vi "LabviewChat.vi"() -> ()   [LabVIEW 2015]
panel:
  out "error 2":errorcluster
  in  "Their IP Address":string
  in  "Receive Port":u16=20090
  in  "Send Port":u16=20090
  in  "Send":bool
  in  "Chat In":string
  out "Chat Out Buffer":string
  out "Chat In Buffer":string
  in  "User Name":string
  out "Chat":string
  out "error out":errorcluster
  in  "stop":bool
  in  "Your IP Address":string
  # "10.2.166.30"
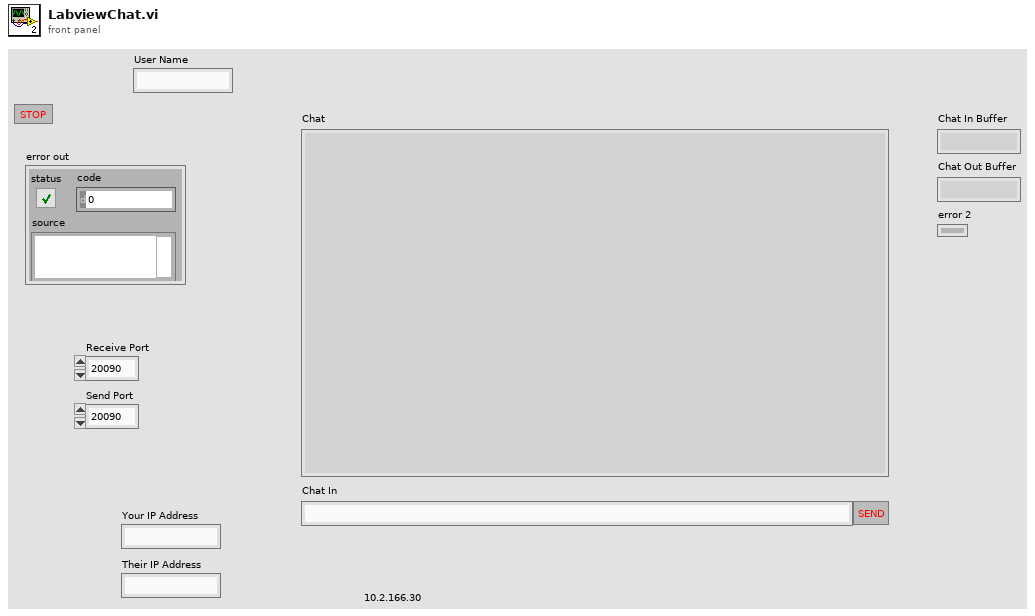
[diagram p1: front panel]
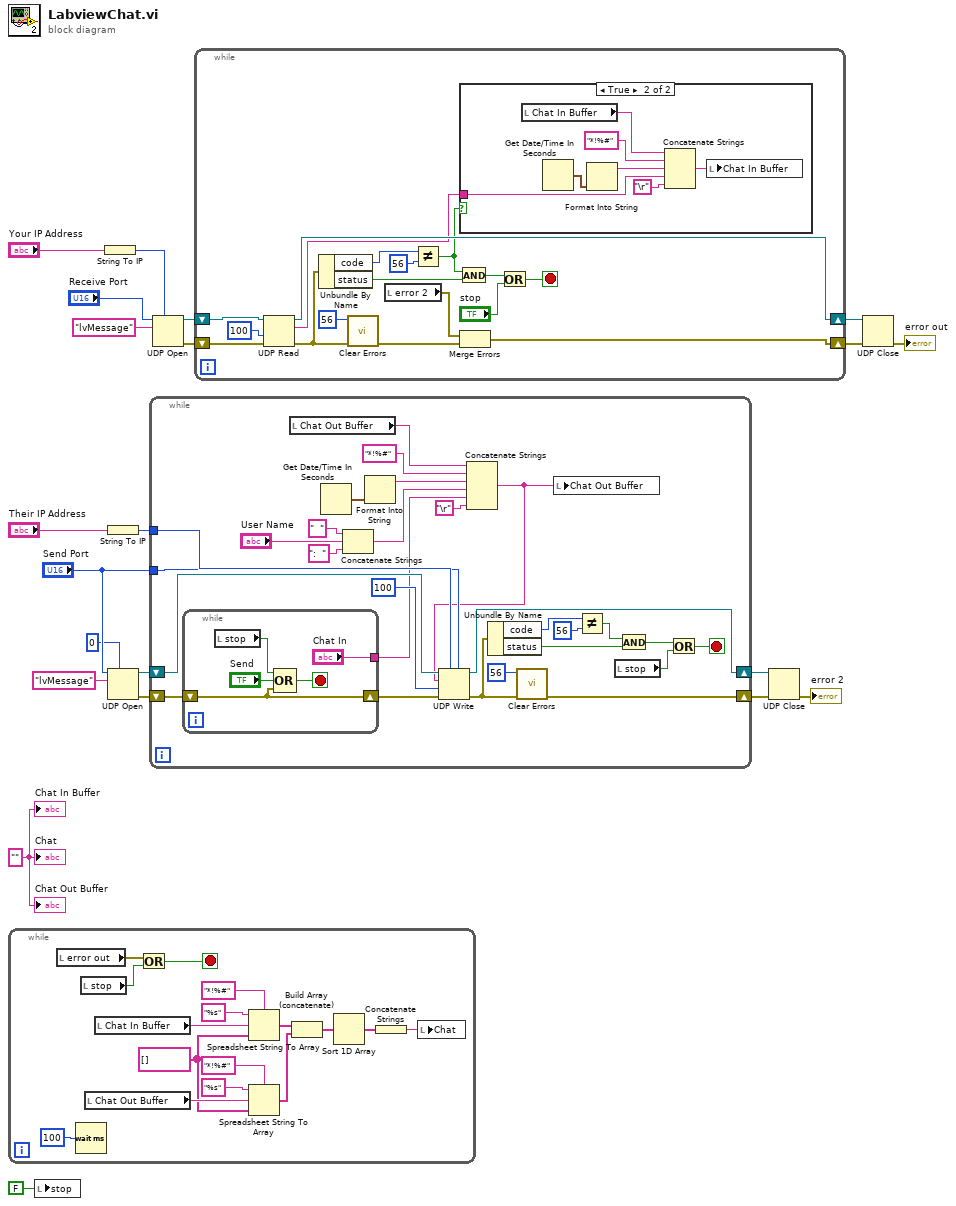
[diagram p0: block diagram]
diagram:
  w8 = "" ("service name")
  n1 = while {
    stop <- w22 stop-if-true
    w25 = string[] []
    n2 = local read "error out"() -> (w24:errorcluster)
    n3 = Wait (ms)(milliseconds to wait=u32 100) -> ()  [unwired: 1 out]
    n4 = local read "stop"() -> (w23:bool)
    n5 = local read "Chat Out Buffer"() -> (w26:string)
    n6 = local read "Chat In Buffer"() -> (w36:string)
    n7 = Or(x=w24, y=w23) -> (x .or. y?=w22:bool)
    n8 = Spreadsheet String To Array(delimiter (Tab)="*!%#", format string="%s", spreadsheet string=w36, array type (2D Dbl)=w25) -> (array=w29:string[])
    n9 = Spreadsheet String To Array(delimiter (Tab)="*!%#", format string="%s", spreadsheet string=w26, array type (2D Dbl)=w25) -> (array=w28:string[])
    n10 = Build Array (concatenate)(w29, w28) -> (w27:string[])
    n11 = Sort 1D Array(array=w27) -> (sorted array=w33:string[])
    n12 = Concatenate Strings(w33) -> (w32:string)
    n13 = local write "Chat"(w32) -> ()
  }
  n14 = local write "stop"(FALSE ("stop")) -> ()
  n15 = String To IP(1:"Your IP Address") -> (0:w15:u32)
  n16 = String To IP(1:"Their IP Address") -> (0:w2:u32)
  n17 = UDP Open(7:u32 0 ("net address"), 10:"lvMessage" ("service name"), 11:"Send Port") -> (port=w10:refnum<k16>, 0:w13:errorcluster)  [unwired: 2 in, 1 out]
  n18 = while {
    shift-right: [w40] -> w12
    shift-left: w13 -> [w53]
    shift-right: [w51] -> w11
    shift-left: w10 -> [w65]
    tunnel: w2 -> [w52]
    tunnel: "Send Port" -> [w39]
    stop <- w61 stop-if-true
    n19 = while {
      tunnel: ["Chat In"] -> w45
      shift-right: [w66] -> w54
      shift-left: w53 -> [w66]
      stop <- w67 stop-if-true
      n20 = local read "stop"() -> (w68:bool)
      n21 = Compound Arithmetic op=OR(w68, "Send", w66) -> (w67:bool)
    }
    n22 = local read "Chat Out Buffer"() -> (w47:string)
    n23 = Get Date/Time In Seconds() -> (seconds since 1Jan1904=w48:timestamp)
    n24 = Concatenate Strings("  " ("string"), "User Name", ":  " ("string")) -> (w41:string)
    n25 = Format Into String(w48) -> (resulting string=w50:string)  [unwired: 3 in, 1 out]
    n26 = Concatenate Strings(w47, "*!%#" ("string"), w50, w41, w45, "\r") -> (w38:string)
    n27 = UDP Write(address=w52, port or service name=w39, connection ID=w65, data in=w38, 8:w54, 9:100 ("timeout ms (25000)")) -> (error out=w58:errorcluster, 3:w51:refnum<k16>)
    n28 = Unbundle By Name(w58) -> ("code"=w64:i32, "status"=w59:bool)
    n29 = call <vilib>:"Clear Errors.vi"("error in (no error)"=w58, "specific error code to clear (0: all)"=56) -> ("error out"=w40:errorcluster)  [unwired: 4 in, 1 out]
    n30 = local write "Chat Out Buffer"(w38) -> ()
    n31 = Not Equal?(x=w64, y=56) -> (x != y?=w56:bool)
    n32 = local read "stop"() -> (w55:bool)
    n33 = And(x=w56, y=w59) -> (x .and. y?=w62:bool)
    n34 = Or(x=w62, y=w55) -> (x .or. y?=w61:bool)
  }
  n35 = UDP Open(7:w15, 10:"lvMessage" ("service name"), 11:"Receive Port") -> (port=w18:refnum<k16>, 0:w21:errorcluster)  [unwired: 2 in, 1 out]
  n36 = while {
    shift-right: [w71] -> w20
    shift-left: w21 -> [w87]
    shift-right: [w86] -> w19
    shift-left: w18 -> [w85]
    stop <- w80 stop-if-true
    n37 = UDP Read(connection ID=w85, timeout ms (25000)=100, 8:w87) -> (data out=w74:string, error out=w77:errorcluster, 3:w86:refnum<k16>)  [unwired: 1 in, 2 out]
    n38 = Unbundle By Name(w77) -> ("code"=w84:i32, "status"=w78:bool)
    n39 = call <vilib>:"Clear Errors.vi"("error in (no error)"=w77, "specific error code to clear (0: all)"=56) -> ("error out"=w72:errorcluster)  [unwired: 4 in, 1 out]
    n40 = local read "error 2"() -> (w73:errorcluster)
    n41 = Not Equal?(x=w84, y=56) -> (x != y?=w75:bool)
    n42 = And(x=w75, y=w78) -> (x .and. y?=w82:bool)
    n43 = case shown="True" w75 {
      tunnel: w74 -> [_ w94]
      frame False {
      }
      frame True {
        n44 = local read "Chat In Buffer"() -> (w90:string)
        n45 = Get Date/Time In Seconds() -> (seconds since 1Jan1904=w91:timestamp)
        n46 = Format Into String(w91) -> (resulting string=w93:string)  [unwired: 3 in, 1 out]
        n47 = Concatenate Strings(w90, "*!%#" ("string"), w93, w94, "\r") -> (w89:string)
        n48 = local write "Chat In Buffer"(w89) -> ()
      }
    }
    n49 = Merge Errors(w73, w72) -> (w71:errorcluster)
    n50 = Or(x=w82, y="stop") -> (x .or. y?=w80:bool)
  }
  n51 = UDP Close(connection ID=w11, 8:w12) -> (error out=→"error 2":errorcluster)  [unwired: 1 out]
  n52 = UDP Close(connection ID=w19, 8:w20) -> (error out=→"error out":errorcluster)  [unwired: 1 out]
  "Chat" <- w8
  "Chat In Buffer" <- w8
  "Chat Out Buffer" <- w8
